vi "CleanUp.vi"(8 "error in (no error)":errorcluster, 11 "Prueba03 in":refnum<class "Prueba03.lvclass">) -> (0 "error out":errorcluster, 3 "Prueba03 out":refnum<class "Prueba03.lvclass">)   [LabVIEW 2019, in "Prueba03.lvclass"]
uses:
  Prueba03.lvclass
  C:/Users/ivan_/Documents/procal/Pruebas/Prueba/Prueba.lvclass
  Prueba/Prueba.lvclass/Prueba.ctl
  Prueba03.lvclass/Prueba03.ctl
  Base de Datos/SQLiteConnector/SQLiteConnection.lvclass
  Prueba/Prueba.lvclass
  Base de Datos/Base de Datos.lvclass
panel:
  out "Tabla_ext":string[][](array[string])
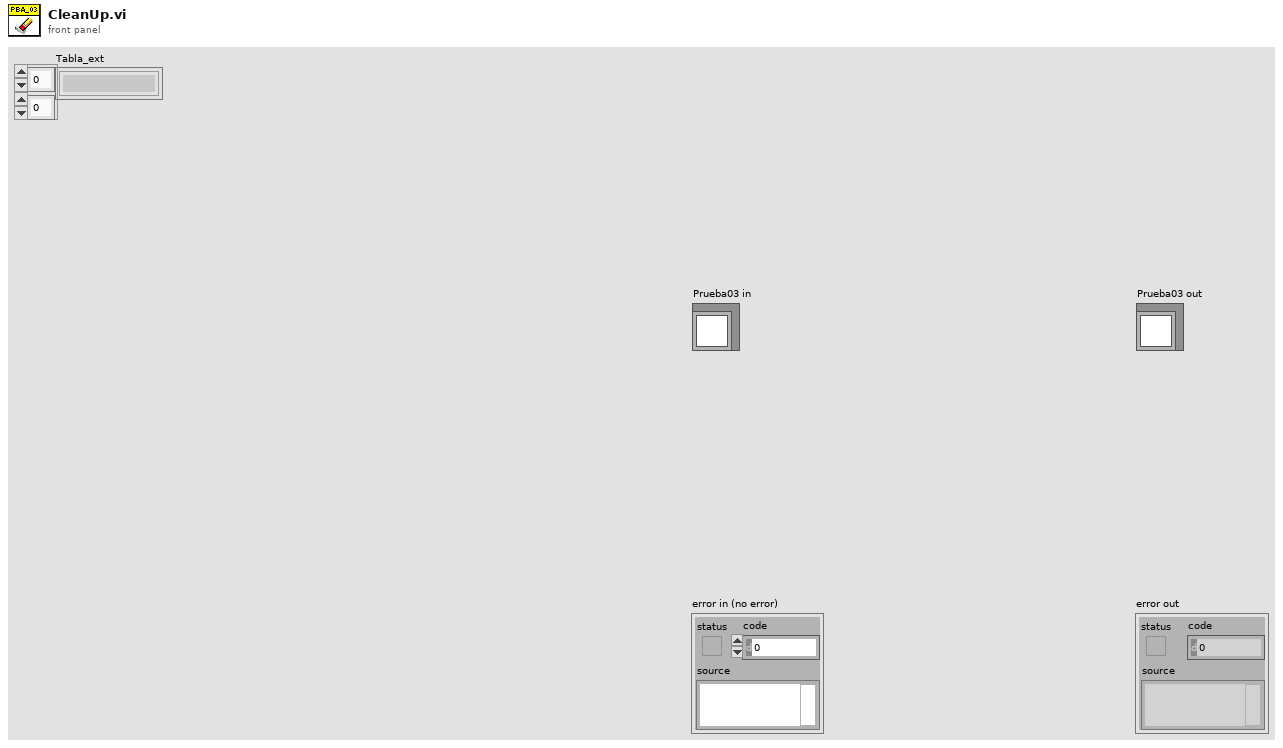
[diagram p1: front panel]
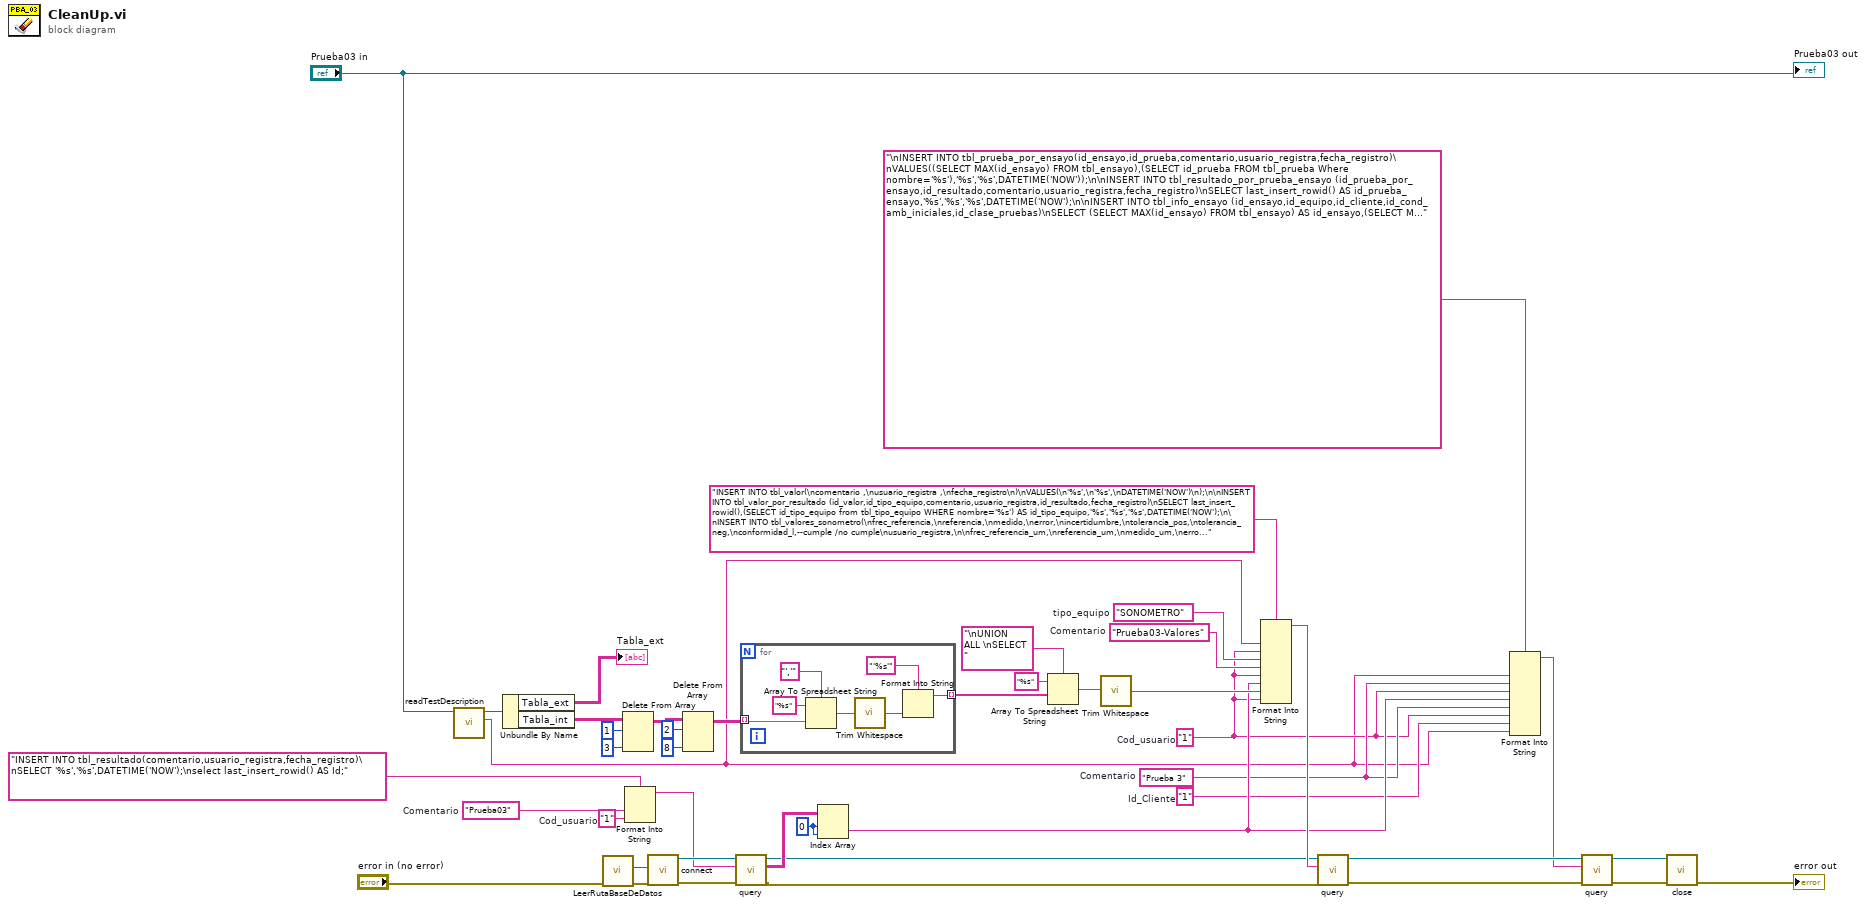
[diagram p0: block diagram]
diagram:
  w19 = "1"  # Id_Cliente
  w20 = "Prueba 3"  # Comentario
  w27 = "SONOMETRO"  # tipo_equipo
  w26 = "Prueba03-Valores"  # Comentario
  w33 = 0 ("index (row)")
  w35 = "1"  # Cod_usuario
  w36 = "Prueba03"  # Comentario
  w18 = "1"  # Cod_usuario
  n1 = call "readTestDescription.vi"("Prueba in"="Prueba03 in") -> ("Test Description"=w7:string, "Prueba out"=w9:refnum<class "Prueba03.lvclass">)  [unwired: 8 in, 1 out]
  n2 = Unbundle By Name(w9) -> ("Tabla_ext"=→"Tabla_ext":string[][], "Tabla_int"=w15:string[][])
  n3 = call "LeerRutaBaseDeDatos.vi"("error in (no error)"="error in (no error)") -> ("error out"=w5:errorcluster, "Database Path"=w4:path)  [unwired: 9 in]
  n4 = Delete From Array(array=w15, length=1, index (col)=3 ("disabled index (col)")) -> (array with subset deleted=w14:string[][])  [unwired: 1 in, 1 out]
  n5 = Format Into String(format string="INSERT INTO tbl_resultado(comentario,usuario_registra,fecha_registro)\nSELECT '%s','%s',DATETIME('NOW');\nselect last_insert_rowid() AS Id;" ("SQL Statement"), w36, w35) -> (resulting string=w34:string)  [unwired: 2 in, 1 out]
  n6 = call "connect.vi"("error in (no error)"=w5, "Database Path"=w4) -> ("error out"=w32:errorcluster, "object out"=w38:refnum<class "SQLiteConnection.lvclass">)  [unwired: 8 in]
  n7 = Delete From Array(array=w14, length=2, index (col)=8 ("disabled index (col)")) -> (array with subset deleted=w11:string[][])  [unwired: 1 in, 1 out]
  n8 = call "query.vi"("error in (no error)"=w32, "SQL Statement"=w34, "object in"=w38) -> ("error out"=w29:errorcluster, "result"=w31:string[][], "object out"=w30:refnum<class "SQLiteConnection.lvclass">)  [unwired: 5 in, 1 out]
  n9 = for {
    tunnel: w11 -> [w51] mode=indexing
    tunnel: [w47] -> w42 mode=indexing
    n10 = Array To Spreadsheet String(delimiter (Tab)="','", array=w51, 3:"%s" ("format string")) -> (spreadsheet string=w46:string)
    n11 = call <vilib>:"Trim Whitespace.vi"("string"=w46) -> ("trimmed string"=w45:string)  [unwired: 1 in]
    n12 = Format Into String(format string="'%s'", w45) -> (resulting string=w47:string)  [unwired: 2 in, 1 out]
  }
  n13 = Index Array(array=w31, index (row)=w33, index (col)=w33) -> (element=w21:string)
  n14 = Array To Spreadsheet String(delimiter (Tab)="\nUNION ALL \nSELECT ", array=w42, 3:"%s" ("format string")) -> (spreadsheet string=w41:string)
  n15 = call <vilib>:"Trim Whitespace.vi"("string"=w41) -> ("trimmed string"=w28:string)  [unwired: 1 in]
  n16 = Format Into String(format string="INSERT INTO tbl_valor(\ncomentario ,\nusuario_registra ,\nfecha_registro\n)\nVALUES(\n'%s',\n'%s',\nDATETIME('NOW')\n);\n\nINSERT INTO tbl_valor_por_resultado (id_valor,id_tipo_equipo,comentario,usuario_registra,id_resultado,fecha_registro)\nSELECT last_insert_rowid(),(SELECT id_tipo_equipo from tbl_tipo_equipo WHERE nombre='%s') AS id_tipo_equipo,'%s','%s','%s',DATETIME('NOW');\n\nINSERT INTO tbl_valores_sonometro(\nfrec_referencia,\nreferencia,\nmedido,\nerror,\nincertidumbre,\ntolerancia_pos,\ntolerancia_neg,\nconformidad_l,--cumple /no cumple\nusuario_registra,\n\nfrec_referencia_um,\nreferencia_um,\nmedido_um,\nerror_um,\nincertidumbre_um,\ntolerancia_pos_um,\ntolerancia_neg_um,\n\nid_valor,\nfecha_registro\n)\nSELECT * FROM(\nSELECT %s\n) AS T\nINNER JOIN\n(SELECT %s AS usuario,'Hz','dB','dB','dB','dB','dB','dB',(SELECT MAX(id_valor) FROM tbl_valor) AS id_valor,DATETIME('NOW') fecha ) AS F;\n", w7, w18, w27, w26, w18, w21, w28, w18) -> (resulting string=w39:string)  [unwired: 2 in, 1 out]
  n17 = call "query.vi"("error in (no error)"=w29, "SQL Statement"=w39, "object in"=w30) -> ("error out"=w24:errorcluster, "object out"=w25:refnum<class "SQLiteConnection.lvclass">)  [unwired: 5 in, 2 out]
  n18 = Format Into String(format string="\nINSERT INTO tbl_prueba_por_ensayo(id_ensayo,id_prueba,comentario,usuario_registra,fecha_registro)\nVALUES((SELECT MAX(id_ensayo) FROM tbl_ensayo),(SELECT id_prueba FROM tbl_prueba Where nombre='%s'),'%s','%s',DATETIME('NOW'));\n\nINSERT INTO tbl_resultado_por_prueba_ensayo (id_prueba_por_ensayo,id_resultado,comentario,usuario_registra,fecha_registro)\nSELECT last_insert_rowid() AS id_prueba_ensayo,'%s','%s','%s',DATETIME('NOW');\n\nINSERT INTO tbl_info_ensayo (id_ensayo,id_equipo,id_cliente,id_cond_amb_iniciales,id_clase_pruebas)\nSELECT (SELECT MAX(id_ensayo) FROM tbl_ensayo) AS id_ensayo,(SELECT MAX(id_equipo) FROM tbl_equipo) AS id_equipo,'%s' AS id_cliente,(SELECT MAX(id_cond_amb_iniciales) FROM tbl_cond_amb_iniciales) AS id_cond_amb_iniciales,\n(SELECT id_clase_prueba FROM tbl_clase_prueba WHERE id_clase=(SELECT id_clase FROM tbl_equipo ORDER BY id_equipo DESC LIMIT 1)  AND id_prueba=(SELECT id_prueba FROM tbl_prueba Where nombre='%s')) AS id_clase_pruebas;\n", w7, w20, w18, w21, w20, w18, w19, w7) -> (resulting string=w22:string)  [unwired: 2 in, 1 out]
  n19 = call "query.vi"("error in (no error)"=w24, "SQL Statement"=w22, "object in"=w25) -> ("error out"=w3:errorcluster, "object out"=w1:refnum<class "SQLiteConnection.lvclass">)  [unwired: 5 in, 2 out]
  n20 = call-dynamic "close.vi"("error in (no error)"=w3, "object in"=w1) -> ("error out"=→"error out":errorcluster)  [unwired: 8 in, 1 out]
  "Prueba03 out" <- "Prueba03 in"
